vi "Test - Add  Property (Numeric).vi"() -> ()   [LabVIEW 2020, in "JSON Schema Generator.lvlib"]
uses:
  <vilib>/JDP Science/JSONtext/LVClass Serializer/JSONtext LVClass Serializer.lvclass
  JSON Schema Generator.lvlib
  <vilib>/addons/_JKI Toolkits/Caraya/classes/Test/Test.lvclass
  <vilib>/addons/_JKI Toolkits/Caraya/classes/Assert/Assert.lvclass
  <vilib>/JDP Science/JSONtext/JSONtext.lvlib
  <vilib>/addons/_JKI Toolkits/Caraya/classes/Assert/Assert Equal Value_Variant.vi
  <vilib>/addons/_JKI Toolkits/Caraya/classes/Assert/Assert Not Error.vi
  <vilib>/addons/_JKI Toolkits/Caraya/classes/Assert/Assert True.vi
  b87f8c03-b0de-4ca0-8354-f7deaa4f33da.vi
  cb6f855b-e6a2-4a07-8021-4495e1c2a4b3.vi
  <vilib>/addons/_JKI Toolkits/Caraya/classes/Assert/Assert False.vi
  090ee0ff-61c6-4352-aefa-74a0241d7d1e.vi
panel:
  in  "Numeric":dbl=534.0
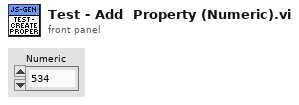
[diagram p1: front panel]
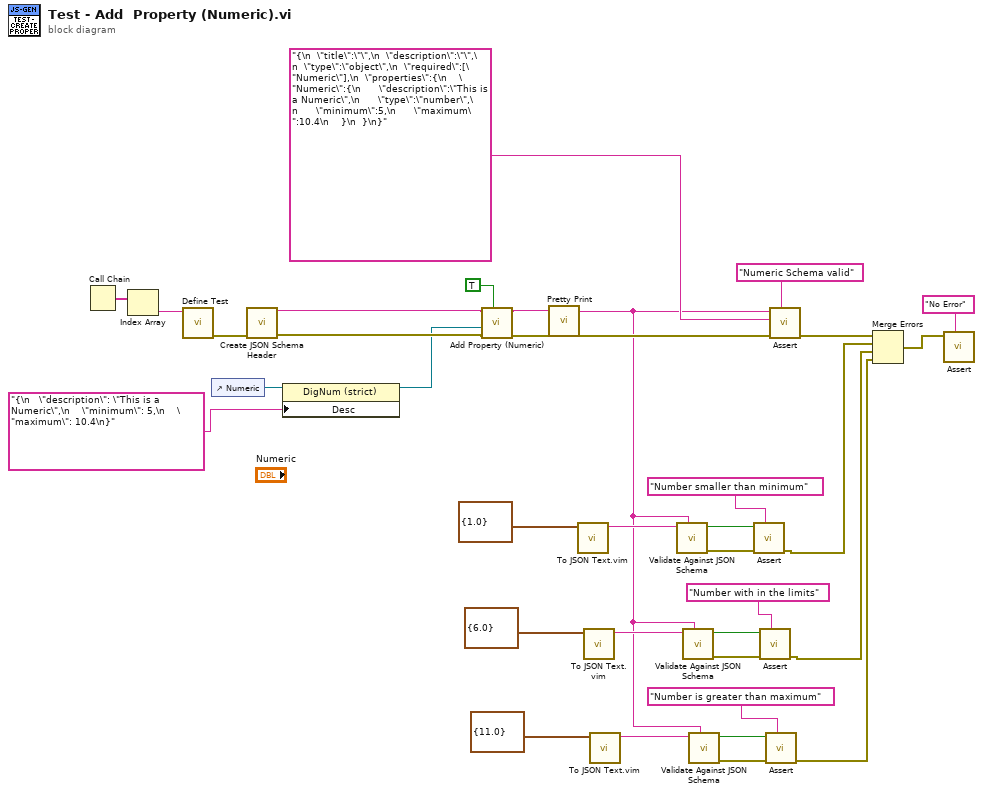
[diagram p0: block diagram]
diagram:
  n1 = Call Chain() -> (call chain=w36:string[])
  n2 = Index Array(array=w36) -> (element=w35:string)  [unwired: 1 in]
  n3 = call <vilib>:"Define Test.vi"("Label (VI Title)"=w35) -> ("error out"=w30:errorcluster)  [unwired: 9 in, 1 out]
  n4 = control-ref of="Numeric"() -> (w22:refnum<vi>)
  n5 = call "Create JSON Schema Header.vi"("error in (no error)"=w30) -> ("error out"=w25:errorcluster, "JSON Schema out"=w27:string)  [unwired: 9 in]
  n6 = property on="Property Node" class="DigNum (strict)"(reference=w22, "Desc"="{\n   \"description\": \"This is a Numeric\",\n    \"minimum\": 5,\n    \"maximum\": 10.4\n}" ("Description")) -> (reference out=w21:refnum<vi>)  [unwired: 1 in, 1 out]
  n7 = call "Add Property (Numeric).vi"("Required?"=TRUE, "error in (no error)"=w25, "Numeric In"=w21, "JSON Schema in"=w27) -> ("error out"=w24:errorcluster, "JSON SChema out"=w26:string)  [unwired: 6 in]
  n8 = call <vilib>:"Pretty Print.vi"("error in (no error)"=w24, "JSON"=w26) -> ("error out"=w29:errorcluster, "<JSON>"=w2:string)  [unwired: 7 in, 1 out]
  n9 = call "To JSON Text.vim"("Anything"=cluster{"Numeric":dbl} {"Numeric"=1.0}) -> ("<JSON>"=w18:string)  [unwired: 9 in, 1 out]
  n10 = call "To JSON Text.vim"("Anything"=cluster{"Numeric":dbl} {"Numeric"=6.0}) -> ("<JSON>"=w10:string)  [unwired: 9 in, 1 out]
  n11 = call "To JSON Text.vim"("Anything"=cluster{"Numeric":dbl} {"Numeric"=11.0}) -> ("<JSON>"=w6:string)  [unwired: 9 in, 1 out]
  n12 = call <vilib>:"Validate Against JSON Schema.vi"("JSON Schema"=w2, "JSON"=w18) -> ("error out"=w15:errorcluster, "Invalid"=w16:bool)  [unwired: 5 in, 3 out]
  n13 = call <vilib>:"Validate Against JSON Schema.vi"("JSON Schema"=w2, "JSON"=w10) -> ("error out"=w13:errorcluster, "Invalid"=w12:bool)  [unwired: 5 in, 3 out]
  n14 = call <vilib>:"Validate Against JSON Schema.vi"("JSON Schema"=w2, "JSON"=w6) -> ("error out"=w3:errorcluster, "Invalid"=w4:bool)  [unwired: 5 in, 3 out]
  n15 = call-poly <vilib>:"Assert.vi"("Label"="Number smaller than minimum", "error in (no error)"=w15, "True?"=w16) -> ("error out"=w14:errorcluster)  [unwired: 7 in, 1 out]
  n16 = call-poly <vilib>:"Assert.vi"("Label"="Number with in the limits", "error in (no error)"=w13, "False?"=w12) -> ("error out"=w8:errorcluster)  [unwired: 7 in, 1 out]
  n17 = call-poly <vilib>:"Assert.vi"("Label"="Number is greater than maximum", "error in (no error)"=w3, "True?"=w4) -> ("error out"=w1:errorcluster)  [unwired: 7 in, 1 out]
  n18 = call-poly <vilib>:"Assert.vi"("Label"="Numeric Schema valid", "error in (no error)"=w29, "Actual"="{\n  \"title\":\"\",\n  \"description\":\"\",\n  \"type\":\"object\",\n  \"required\":[\"Numeric\"],\n  \"properties\":{\n    \"Numeric\":{\n      \"description\":\"This is a Numeric\",\n      \"type\":\"number\",\n      \"minimum\":5,\n      \"maximum\":10.4\n    }\n  }\n}", "Expected"=w2) -> ("error out"=w33:errorcluster)  [unwired: 6 in, 1 out]
  n19 = Merge Errors(w33, w14, w8, w1) -> (w31:errorcluster)
  n20 = call-poly <vilib>:"Assert.vi"("Label"="No Error", "Not Error?"=w31) -> ()  [unwired: 8 in, 2 out]
